vi "Find Default Events Path.vi"(8 "error in":errorcluster, 10 "Event":string, 11 "DQMH Library Ref":refnum<vi>) -> (0 "error out":errorcluster, 3 "Event Path":path)   [LabVIEW 2019, in "Panther Dashboard.lvlib"]
uses:
  Panther Dashboard.lvlib
  <vilib>/Utility/error.llb/Error Cluster From Error Code.vi
  <vilib>/ErrorRing/Error Ring.xnode
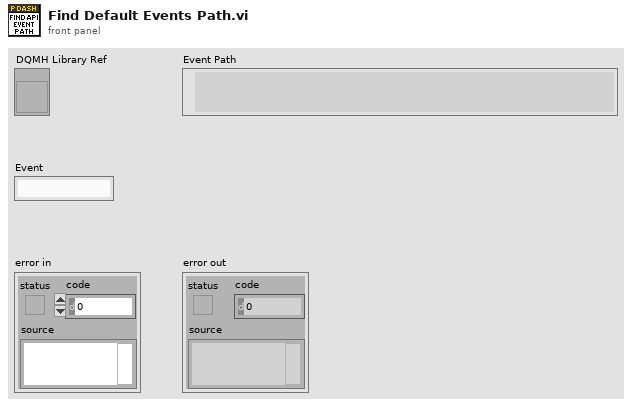
[diagram p1: front panel]
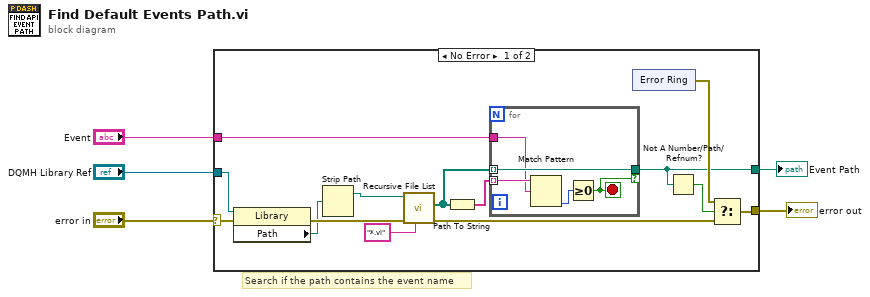
[diagram p0: block diagram]
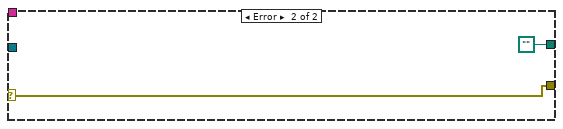
[diagram p2: hidden frame]
diagram:
  # "Search if the path contains the event name"
  n1 = case shown="No Error" "error in" {
    selector: "error in" -> [w15 w31]
    tunnel: [w9 path ""] -> w3
    tunnel: [w17 w31] -> w4
    tunnel: "DQMH Library Ref" -> [w10 _]
    tunnel: "Event" -> [w7 _]
    frame No Error {
      n2 = property class="Library"(reference=w10, error in=w15) -> (error out=w16:errorcluster, "Path"=w11:path)  [unwired: 1 out]
      n3 = Strip Path(path=w11) -> (stripped path=w12:path)  [unwired: 1 out]
      n4 = call <vilib>:"Recursive File List.vi"("pattern"="*.vi", "error in (no error)"=w16, "Folder Path"=w12) -> ("error out"=w18:errorcluster, "All Files in Dir"=w13:path[])  [unwired: 4 in, 3 out]
      n5 = Path To String(path=w13) -> (string=w6:string[])
      n6 = for {
        tunnel: w6 -> [w28] mode=indexing
        tunnel: w13 -> [w29] mode=indexing
        tunnel: [w29] -> w9 if=w26
        tunnel: w7 -> [w25]
        stop <- w26 stop-if-true
        n7 = Match Pattern(string=w28, regular expression=w25) -> (offset past match=w27:i32)  [unwired: 1 in, 3 out]
        n8 = Greater Or Equal To 0?(x=w27) -> (x >= 0?=w26:bool)
      }
      n9 = xnode "Error Ring"() -> ("error out"=w19:errorcluster)
      n10 = Not A Number/Path/Refnum?(number/path/refnum=w9) -> (NaN/Path/Refnum?=w8:bool)
      n11 = Select(t=w19, s=w8, f=w18) -> (s? t:f=w17:errorcluster)
    }
    frame Error {
    }
  }
  "Event Path" <- w3
  "error out" <- w4
